vi "txtfilewriter (SubVI).vi"(8 "error in (no error)":errorcluster, 10 "String":string, 11 "actual path":path) -> (0 "error out":errorcluster)   [LabVIEW 2017]
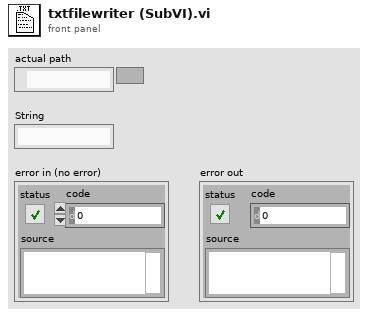
[diagram p1: front panel]
types:
  T1 = enum16{"open", "replace", "create", "open or create", "replace or create", "replace or create with confirmation"}
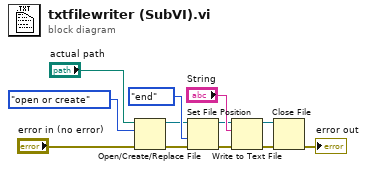
[diagram p0: block diagram]
diagram:
  n1 = Open/Create/Replace File(file path (use dialog)="actual path", error in="error in (no error)", operation (0:open)=T1."open or create") -> (refnum out=w5:refnum<file>, error out=w3:errorcluster)  [unwired: 3 in, 1 out]
  n2 = Set File Position(refnum=w5, from (0:start)=enum16{"start", "end", "current"}."end", error in=w3) -> (refnum out=w8:refnum<file>, error out=w4:errorcluster)  [unwired: 1 in]
  n3 = Write to Text File(file (use dialog)=w8, text="String", error in=w4) -> (refnum out=w1:refnum<file>, error out=w10:errorcluster)  [unwired: 1 in, 1 out]
  n4 = Close File(refnum=w1, error in=w10) -> (error out=→"error out":errorcluster)  [unwired: 1 out]
